vi "Scan Setup.vi"(8 "error in (no error)":errorcluster, 11 "Pulse Gen Basic Scan in":refnum<class "Pulse Gen Basic Scan.lvclass">) -> (0 "error out":errorcluster, 3 "Pulse Gen Basic Scan out":refnum<class "Pulse Gen Basic Scan.lvclass">)   [LabVIEW 2017, in "Pulse Gen Basic Scan.lvclass"]
doc: "Configure the Instrument based on the class member fields. This step comes after the user has closed the \"Scan Setup\" window and before the actual scan -- so instruments are configured with the user's specified settings."
uses:
  Pulse Gen Basic Scan.lvclass
  Scanner/Scanner.lvclass
  Instruments/Utility Classes/Scannable/Scannable.lvclass
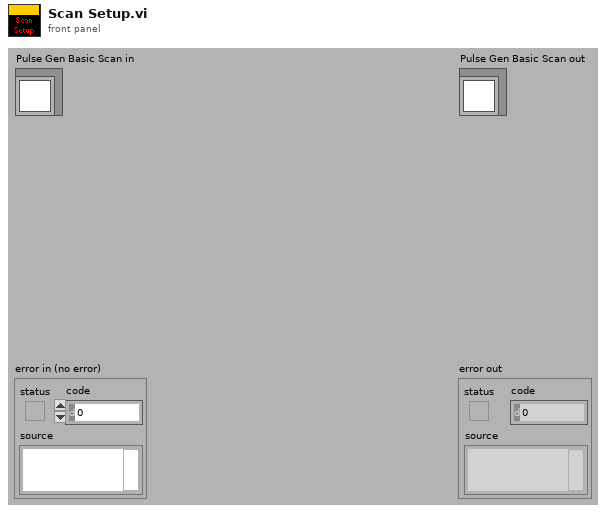
[diagram p1: front panel]
types:
  T1 = enum16{"Internal Oscillator", "Internal PLL", "External Clock "}
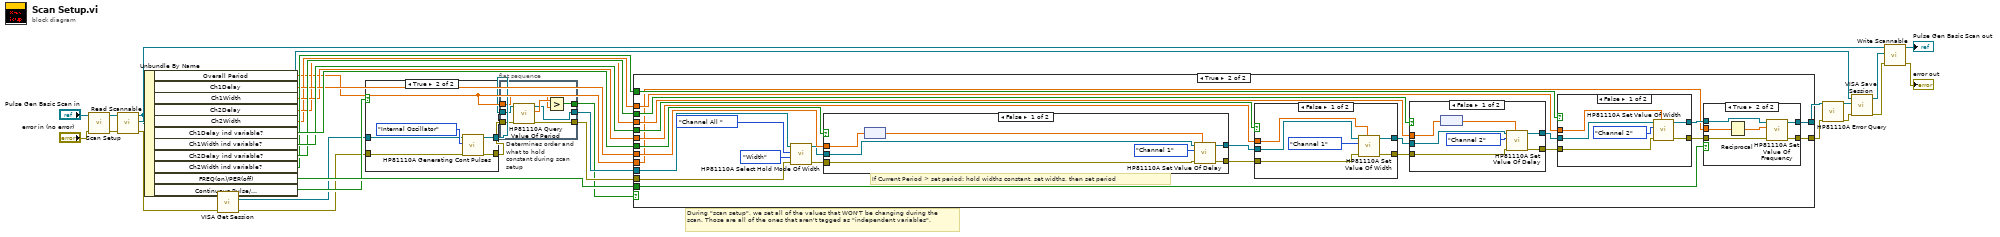
[diagram p0: block diagram]
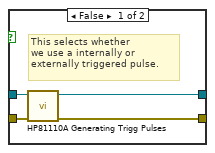
[diagram p2: hidden frame]
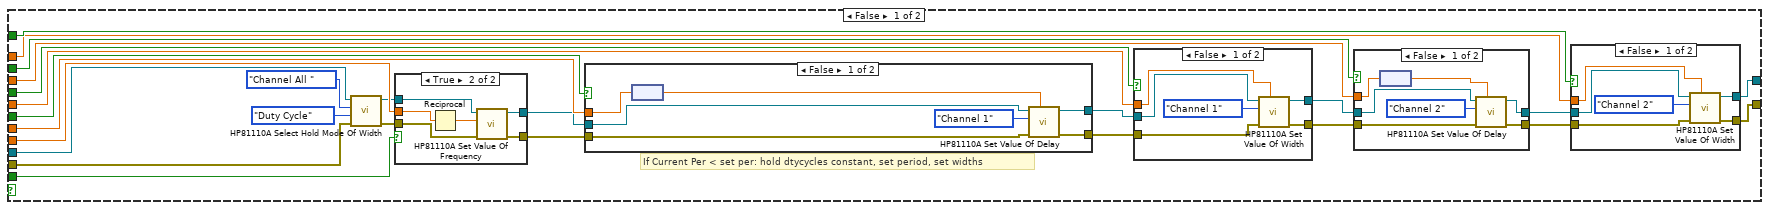
[diagram p3: hidden frame]
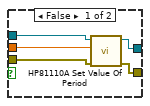
[diagram p4: hidden frame]
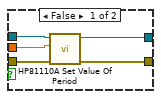
[diagram p9: hidden frame]
diagram:
  # "During \"scan setup\", we set all of the values that WON'T be changing during the scan. Those are all of the ones that aren't tagged as \"independent variables\"."
  n1 = call-parent "Scan Setup.vi"("error in (no error)"="error in (no error)", "Scanner in"="Pulse Gen Basic Scan in") -> ("error out"=w23:errorcluster, "Scanner out"=w24:refnum<class "Pulse Gen Basic Scan.lvclass">)  [unwired: 8 in]
  n2 = call-dynamic "Read Scannable.vi"("error in (no error)"=w23, "Scanner.lvclass in"=w24) -> ("error out"=w21:errorcluster, "Scannable.lvclass"=w22:refnum<class "Scannable.lvclass">, "Scanner.lvclass out"=w18:refnum<class "Pulse Gen Basic Scan.lvclass">)  [unwired: 7 out]
  n3 = Unbundle By Name(w18) -> ("Overall Period"=w6:dbl[unit], "Ch1Delay"=w28:dbl[unit], "Ch1Width"=w27:dbl[unit], "Ch2Delay"=w26:dbl[unit], "Ch2Width"=w25:dbl[unit], "Ch1Delay ind variable?"=w32:bool, "Ch1Width ind variable?"=w31:bool, "Ch2Delay ind variable?"=w30:bool, "Ch2Width ind variable?"=w29:bool, "FREQ(on)/PER(off)"=w10:bool, "Continuous Pulse/ \nExt Triggered Pulse"=w5:bool)
  n4 = call-dynamic "VISA Get Session.vi"("error in (no error)"=w21, "Instrument.lvclass in"=w22) -> ("error out"=w3:errorcluster, "VISA Resource Name"=w4:refnum<visa-resource-name>, "Instrument.lvclass out"=w11:refnum<class "Scannable.lvclass">)  [unwired: 7 out]
  n5 = case shown="True" w5 {
    tunnel: w4 -> [w38 w42]
    tunnel: w3 -> [w37 w41]
    tunnel: [w36 w40] -> w1
    tunnel: [w35 w39] -> w2
    frame False {
      # "This selects whether\nwe use a internally or\nexternally triggered pulse."
      n6 = call "HP81110A Generating Trigg Pulses.vi"("error in (no error)"=w37, "VISA session"=w38) -> ("error out"=w36:errorcluster, "dup VISA session"=w35:refnum<visa-resource-name>)  [unwired: 8 in]
    }
    frame True {
      n7 = call "HP81110A Generating Cont Pulses.vi"("error in (no error)"=w41, "Period Source (0:Internal)"=T1."Internal Oscillator", "VISA session"=w42) -> ("error out"=w40:errorcluster, "dup VISA session"=w39:refnum<visa-resource-name>)  [unwired: 7 in]
    }
  }
  n8 = flat-sequence "Determines order and what to hold\nconstant during scan setup" {
    tunnel: w2 -> [w50]
    tunnel: w1 -> [w49]
    tunnel: [w47] -> w9
    tunnel: [w46] -> w8
    tunnel: [w45] -> w7
    tunnel: w6 -> [w44]
    frame #0 {
      n9 = call "HP81110A Query Value Of Period.vi"("error in (no error)"=w49, "VISA session"=w50) -> ("error out"=w46:errorcluster, "Period Value"=w48:dbl[unit], "dup VISA session"=w47:refnum<visa-resource-name>)  [unwired: 7 in]
      n10 = Greater?(x=w48, y=w44) -> (0:w45:bool)
    }
  }
  n11 = case shown="True" w7 {
    tunnel: w32 -> [w76 w146]
    tunnel: w31 -> [w75 w145]
    tunnel: w30 -> [w74 w143]
    tunnel: w29 -> [w73 w141]
    tunnel: w28 -> [w66 w147]
    tunnel: w27 -> [w65 w144]
    tunnel: w26 -> [w64 w142]
    tunnel: w25 -> [w63 w140]
    tunnel: [w62 w130] -> w14
    tunnel: [w61 w131] -> w12
    tunnel: w6 -> [w60 w129]
    tunnel: w8 -> [w55 w126]
    tunnel: w9 -> [w56 w127]
    tunnel: w10 -> [w57 w128]
    frame False {
      # "If Current Per < set per: hold dtycycles constant, set period, set widths"
      n12 = call "HP81110A Select Hold Mode Of Width.vi"("error in (no error)"=w55, "Width Hold Mode (0:Width)"=enum16{"Width", "Duty Cycle", "Trailing Delay"}."Duty Cycle", "Channel (1:Channel 1)"=enum16{"Channel All ", "Channel 1", "Channel 2"}."Channel All ", "VISA session"=w56) -> ("error out"=w51:errorcluster, "dup VISA session"=w52:refnum<visa-resource-name>)  [unwired: 6 in]
      n13 = case shown="True" w57 {
        tunnel: w60 -> [w80 w86]
        tunnel: w51 -> [w79 w85]
        tunnel: [w78 w84] -> w59
        tunnel: w52 -> [w81 w83]
        tunnel: [w77 w82] -> w58
        frame False {
          n14 = call "HP81110A Set Value Of Period.vi"("error in (no error)"=w79, "Period Value"=w80, "VISA session"=w81) -> ("error out"=w78:errorcluster, "dup VISA session"=w77:refnum<visa-resource-name>)  [unwired: 7 in]
        }
        frame True {
          n15 = Reciprocal(x=w86) -> (1/x=w87:dbl[unit])
          n16 = call "HP81110A Set Value Of Frequency.vi"("error in (no error)"=w85, "Frequency Value"=w87, "VISA session"=w83) -> ("error out"=w84:errorcluster, "dup VISA session"=w82:refnum<visa-resource-name>)  [unwired: 7 in]
        }
      }
      n17 = case shown="False" w76 {
        tunnel: w58 -> [w119 w121]
        tunnel: [w118 w121] -> w72
        tunnel: w59 -> [w117 w120]
        tunnel: [w116 w120] -> w69
        tunnel: w66 -> [w114 _]
        frame False {
          n18 = node(w114) -> (w113:dbl)
          n19 = call "HP81110A Set Value Of Delay.vi"("Delay Value (0.0)"=w113, "error in (no error)"=w117, "Channel (1:Channel 1)"=enum16{"Channel All ", "Channel 1", "Channel 2"}."Channel 1", "VISA session"=w119) -> ("error out"=w116:errorcluster, "dup VISA session"=w118:refnum<visa-resource-name>)  [unwired: 6 in]
        }
        frame True {
        }
      }
      n20 = case shown="False" w75 {
        tunnel: w72 -> [w110 w112]
        tunnel: [w109 w112] -> w71
        tunnel: w69 -> [w108 w111]
        tunnel: [w107 w111] -> w68
        tunnel: w65 -> [w105 _]
        frame False {
          n21 = call "HP81110A Set Value Of Width.vi"("Width Value (100.0E-9)"=w105, "error in (no error)"=w108, "Channel (1:Channel 1)"=enum16{"Channel All ", "Channel 1", "Channel 2"}."Channel 1", "VISA session"=w110) -> ("error out"=w107:errorcluster, "dup VISA session"=w109:refnum<visa-resource-name>)  [unwired: 6 in]
        }
        frame True {
        }
      }
      n22 = case shown="False" w74 {
        tunnel: w71 -> [w102 w104]
        tunnel: [w101 w104] -> w70
        tunnel: w68 -> [w100 w103]
        tunnel: [w99 w103] -> w67
        tunnel: w64 -> [w97 _]
        frame False {
          n23 = node(w97) -> (w96:dbl)
          n24 = call "HP81110A Set Value Of Delay.vi"("Delay Value (0.0)"=w96, "error in (no error)"=w100, "Channel (1:Channel 1)"=enum16{"Channel All ", "Channel 1", "Channel 2"}."Channel 2", "VISA session"=w102) -> ("error out"=w99:errorcluster, "dup VISA session"=w101:refnum<visa-resource-name>)  [unwired: 6 in]
        }
        frame True {
        }
      }
      n25 = case shown="False" w73 {
        tunnel: w70 -> [w93 w94]
        tunnel: w67 -> [w92 w95]
        tunnel: [w91 w95] -> w62
        tunnel: w63 -> [w89 _]
        tunnel: [w88 w94] -> w61
        frame False {
          n26 = call "HP81110A Set Value Of Width.vi"("Width Value (100.0E-9)"=w89, "error in (no error)"=w92, "Channel (1:Channel 1)"=enum16{"Channel All ", "Channel 1", "Channel 2"}."Channel 2", "VISA session"=w93) -> ("error out"=w91:errorcluster, "dup VISA session"=w88:refnum<visa-resource-name>)  [unwired: 6 in]
        }
        frame True {
        }
      }
    }
    frame True {
      # "If Current Period > set period: hold widths constant, set widths, then set period"
      n27 = call "HP81110A Select Hold Mode Of Width.vi"("error in (no error)"=w126, "Width Hold Mode (0:Width)"=enum16{"Width", "Duty Cycle", "Trailing Delay"}."Width", "Channel (1:Channel 1)"=enum16{"Channel All ", "Channel 1", "Channel 2"}."Channel All ", "VISA session"=w127) -> ("error out"=w125:errorcluster, "dup VISA session"=w124:refnum<visa-resource-name>)  [unwired: 6 in]
      n28 = case shown="False" w146 {
        tunnel: w124 -> [w190 w192]
        tunnel: [w189 w192] -> w139
        tunnel: w125 -> [w188 w191]
        tunnel: [w187 w191] -> w138
        tunnel: w147 -> [w185 _]
        frame False {
          n29 = node(w185) -> (w184:dbl)
          n30 = call "HP81110A Set Value Of Delay.vi"("Delay Value (0.0)"=w184, "error in (no error)"=w188, "Channel (1:Channel 1)"=enum16{"Channel All ", "Channel 1", "Channel 2"}."Channel 1", "VISA session"=w190) -> ("error out"=w187:errorcluster, "dup VISA session"=w189:refnum<visa-resource-name>)  [unwired: 6 in]
        }
        frame True {
        }
      }
      n31 = case shown="False" w145 {
        tunnel: w139 -> [w181 w183]
        tunnel: [w180 w183] -> w137
        tunnel: w138 -> [w179 w182]
        tunnel: [w178 w182] -> w136
        tunnel: w144 -> [w176 _]
        frame False {
          n32 = call "HP81110A Set Value Of Width.vi"("Width Value (100.0E-9)"=w176, "error in (no error)"=w179, "Channel (1:Channel 1)"=enum16{"Channel All ", "Channel 1", "Channel 2"}."Channel 1", "VISA session"=w181) -> ("error out"=w178:errorcluster, "dup VISA session"=w180:refnum<visa-resource-name>)  [unwired: 6 in]
        }
        frame True {
        }
      }
      n33 = case shown="False" w143 {
        tunnel: w137 -> [w173 w175]
        tunnel: [w172 w175] -> w135
        tunnel: w136 -> [w171 w174]
        tunnel: [w170 w174] -> w134
        tunnel: w142 -> [w168 _]
        frame False {
          n34 = node(w168) -> (w167:dbl)
          n35 = call "HP81110A Set Value Of Delay.vi"("Delay Value (0.0)"=w167, "error in (no error)"=w171, "Channel (1:Channel 1)"=enum16{"Channel All ", "Channel 1", "Channel 2"}."Channel 2", "VISA session"=w173) -> ("error out"=w170:errorcluster, "dup VISA session"=w172:refnum<visa-resource-name>)  [unwired: 6 in]
        }
        frame True {
        }
      }
      n36 = case shown="False" w141 {
        tunnel: w135 -> [w164 w165]
        tunnel: w134 -> [w163 w166]
        tunnel: [w162 w166] -> w132
        tunnel: w140 -> [w160 _]
        tunnel: [w159 w165] -> w133
        frame False {
          n37 = call "HP81110A Set Value Of Width.vi"("Width Value (100.0E-9)"=w160, "error in (no error)"=w163, "Channel (1:Channel 1)"=enum16{"Channel All ", "Channel 1", "Channel 2"}."Channel 2", "VISA session"=w164) -> ("error out"=w162:errorcluster, "dup VISA session"=w159:refnum<visa-resource-name>)  [unwired: 6 in]
        }
        frame True {
        }
      }
      n38 = case shown="True" w128 {
        tunnel: [w152 w157] -> w130
        tunnel: [w151 w156] -> w131
        tunnel: w129 -> [w150 w155]
        tunnel: w133 -> [w149 w154]
        tunnel: w132 -> [w148 w153]
        frame False {
          n39 = call "HP81110A Set Value Of Period.vi"("error in (no error)"=w148, "Period Value"=w150, "VISA session"=w149) -> ("error out"=w152:errorcluster, "dup VISA session"=w151:refnum<visa-resource-name>)  [unwired: 7 in]
        }
        frame True {
          n40 = Reciprocal(x=w155) -> (1/x=w158:dbl[unit])
          n41 = call "HP81110A Set Value Of Frequency.vi"("error in (no error)"=w153, "Frequency Value"=w158, "VISA session"=w154) -> ("error out"=w157:errorcluster, "dup VISA session"=w156:refnum<visa-resource-name>)  [unwired: 7 in]
        }
      }
    }
  }
  n42 = call "HP81110A Error Query.vi"("VISA session"=w12, "error in (no error)"=w14) -> ("dup VISA session"=w13:refnum<visa-resource-name>, "error out"=w15:errorcluster)  [unwired: 10 in, 2 out]
  n43 = call-dynamic "VISA Save Session.vi"("error in (no error)"=w15, "VISA Resource Name"=w13, "Instrument.lvclass in"=w11) -> ("error out"=w20:errorcluster, "Instrument.lvclass out"=w19:refnum<class "Scannable.lvclass">)  [unwired: 7 out]
  n44 = call-dynamic "Write Scannable.vi"("error in (no error)"=w20, "Scannable.lvclass"=w19, "Scanner.lvclass in"=w18) -> ("error out"=→"error out":errorcluster, "Scanner.lvclass out"=→"Pulse Gen Basic Scan out":refnum<class "Pulse Gen Basic Scan.lvclass">)  [unwired: 7 out]
